vi "CRYCompare all  Y_axis units.vi"(11 "Y_axis array in":string[](array[string])) -> (3 "All erqal?":bool)   [LabVIEW 2013]
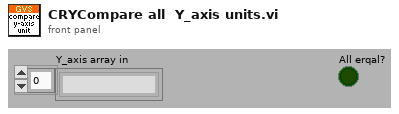
[diagram p1: front panel]
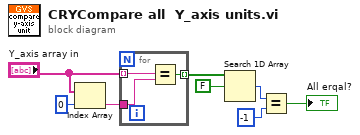
[diagram p0: block diagram]
diagram:
  n1 = Index Array(array="Y_axis array in", index=0) -> (element=w7:string)
  n2 = for {
    tunnel: "Y_axis array in" -> [w11] mode=indexing
    tunnel: w7 -> [w10]
    tunnel: [w9] -> w6 mode=indexing
    n3 = Equal?(x=w11, y=w10) -> (x = y?=w9:bool)
  }
  n4 = Search 1D Array(1D array=w6, element=FALSE) -> (index of element=w4:i32)  [unwired: 1 out]
  n5 = Equal?(x=w4, y=-1) -> (x = y?=→"All erqal?":bool)
